vi "Write_fit_data.vi"(4 "dset name":string, 5 "error in":errorcluster, 6 "fit attribs":variant[](array[variant]), 7 "fit_params":T1(array[cluster]), 8 "ref in":i32) -> (0 "error out":errorcluster, 3 "ref out":i32)   [LabVIEW 2010]
uses:
  <vilib>/addons/h5labview2/attrib/H5Awrite.llb/H5Awrite.xnode
  <vilib>/addons/h5labview2/base/H5Equery.vi
  <vilib>/addons/h5labview2/h5labview.lib
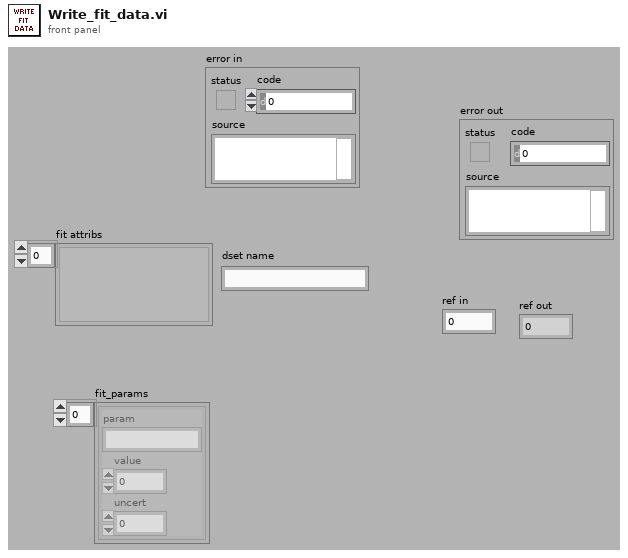
[diagram p1: front panel]
types:
  T1 = cluster{"param":string, "value":dbl, "uncert":dbl}[]
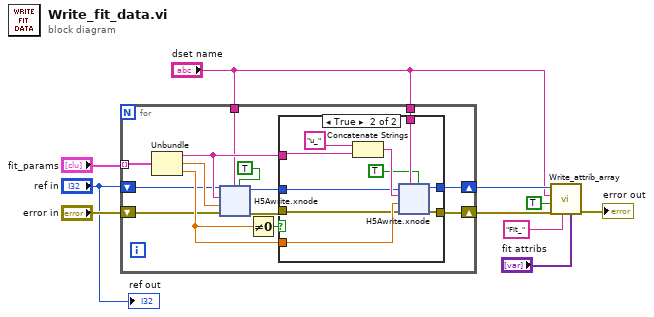
[diagram p0: block diagram]
diagram:
  n1 = for {
    tunnel: "fit_params" -> [w24] mode=indexing
    shift-right: [w20] -> w5
    shift-left: "error in" -> [w11]
    shift-right: [w21] -> w6
    shift-left: "ref in" -> [w12]
    tunnel: "dset name" -> [w16]
    tunnel: "dset name" -> [w19]
    n2 = Unbundle(w24) -> ("param"=w18:string, "value"=w17:dbl, "uncert"=w22:dbl)
    n3 = xnode "H5Awrite.xnode"("replace? (T)"=TRUE ("overwrite?"), "object name"=w16, "error in (no error)"=w11, "data"=w17, "attrib name"=w18, "ref in"=w12) -> ("error out"=w14:errorcluster, "ref out"=w15:i32)  [unwired: 1 in, 1 out]
    n4 = Not Equal To 0?(x=w22) -> (x != 0?=w23:bool)
    n5 = case shown="True" w23 {
      tunnel: w14 -> [w42 w45]
      tunnel: w15 -> [w43 w46]
      tunnel: [w43 w50] -> w21
      tunnel: w18 -> [_ w53]
      tunnel: w22 -> [_ w47]
      tunnel: [w42 w51] -> w20
      tunnel: w19 -> [_ w49]
      frame False {
      }
      frame True {
        n6 = Concatenate Strings("u_" ("string"), w53) -> (w48:string)
        n7 = xnode "H5Awrite.xnode"("replace? (T)"=TRUE ("overwrite?"), "object name"=w49, "error in (no error)"=w45, "data"=w47, "attrib name"=w48, "ref in"=w46) -> ("error out"=w51:errorcluster, "ref out"=w50:i32)  [unwired: 1 in, 1 out]
      }
    }
  }
  n8 = call <userlib>:"Write_attrib_array.vi"("attribs"="fit attribs", "prefix"="Fit_", "error in (no error)"=w5, "overwrite?"=TRUE, "obj_name"="dset name", "ref"=w6) -> ("error out"=→"error out":errorcluster)  [unwired: 2 in, 1 out]
  "ref out" <- "ref in"
